vi "indicater.vi"() -> ()   [LabVIEW 2012]
panel:
  in  "stop":bool
  out "K":i16
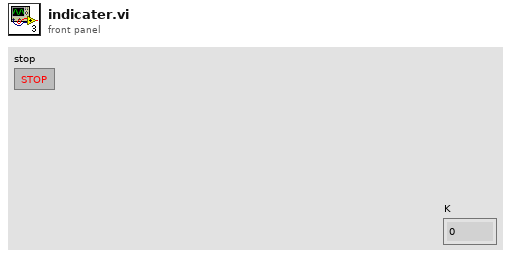
[diagram p1: front panel]
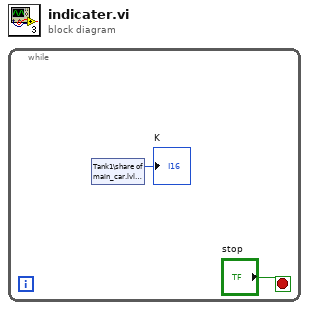
[diagram p0: block diagram]
diagram:
  n1 = while {
    stop <- "stop" stop-if-true
    n2 = shared-variable "Tank1\\share of main_car.lvlib\\K"() -> (→"K":i16)  [unwired: 1 in, 1 out]
  }
